vi "Fetch Control Method Info.vi"(6 "Parser Settings":T1, 8 "Error in":errorcluster caption="Error in (no error)", 10 "Dispatch (None)":T4, 11 "VI in":refnum<vi>) -> (0 "Error out":errorcluster, 3 "Method Spec Cluster":T5)   [LabVIEW 2023, in "VIDoc Parsing.lvlib"]
uses:
  VIDoc Parsing.lvlib
  TypeDefs/Method Spec Cluster.ctl
  TypeDefs/VI Type Extended Enum.ctl
  <vilib>/picture/picture.llb/imagedata.ctl
  TypeDefs/Class Dispatch Type Enum.ctl
  TypeDefs/Controls Info Cluster.ctl
  <vilib>/Utility/miscctls.llb/LVKeyTypeDef.ctl
  <vilib>/Utility/miscctls.llb/LVPointTypeDef.ctl
  Structure Reporter/Tree Cluster.ctl
  Settings/Parser Settings/Parser Settings Cluster.ctl
  Settings/Parser Settings/Draw Controls Cluster.ctl
  Settings/Parser Settings/Draw Option Enum.ctl
  Structure Reporter/Structure Reporter.lvlib
  Settings/Parser Settings/Parser Settings.lvclass
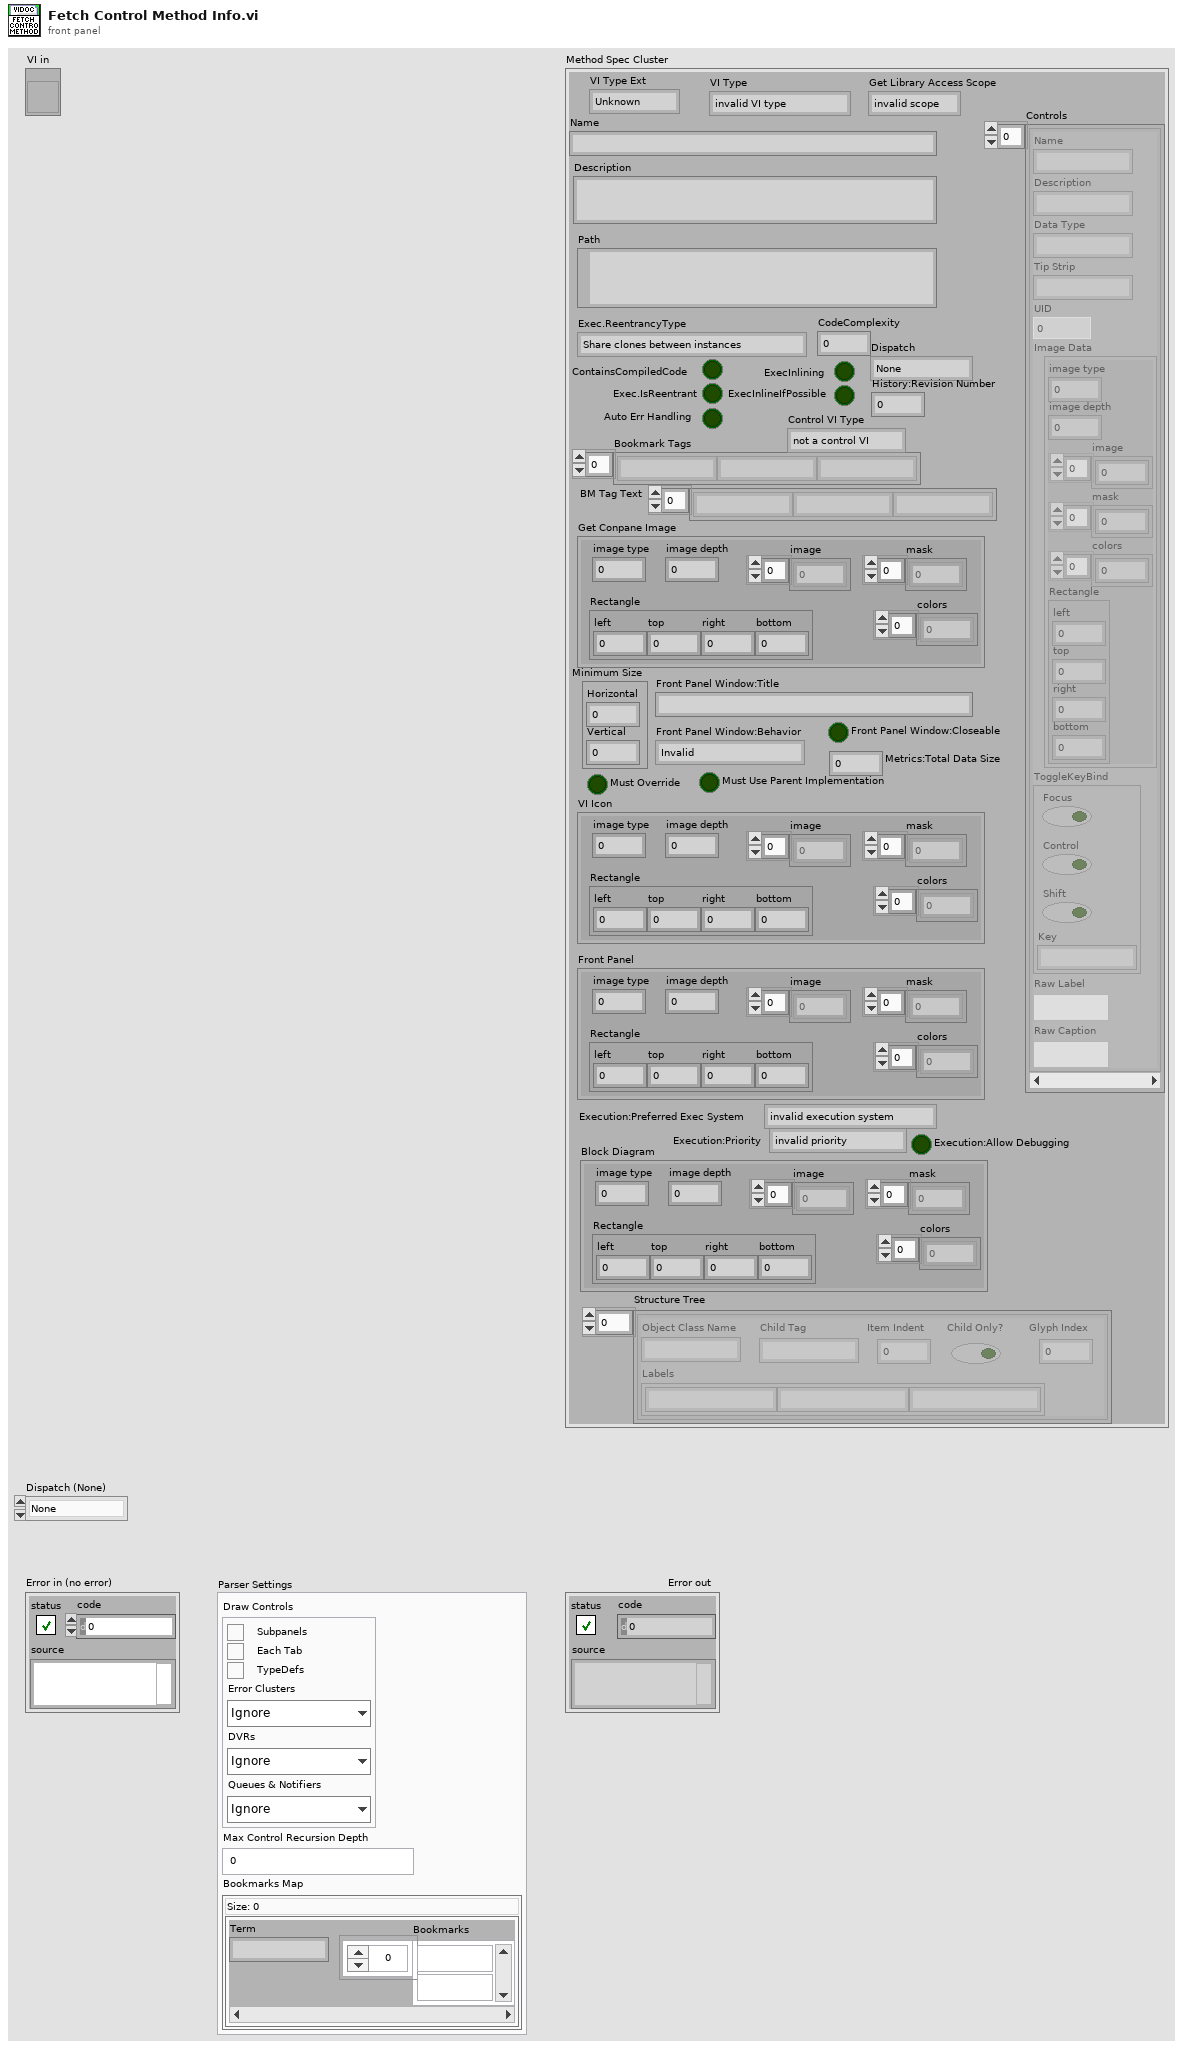
[diagram p1: front panel]
types:
  T1 = typedef "VIDoc Parsing.lvlib/Parser Settings.lvclass/Parser Settings Cluster.ctl" = cluster{"Draw Controls":T2, "Max Control Recursion Depth":i32, "Bookmarks Map":map{string, string[]}}
  T2 = typedef "VIDoc Parsing.lvlib/Parser Settings.lvclass/Draw Controls Cluster.ctl" = cluster{"Subpanels":bool, "Tabs":bool, "TypeDefs":bool, "Error Clusters":T3, "DVRs":T3, "Queues & Notifiers":T3}
  T3 = typedef "VIDoc Parsing.lvlib/Parser Settings.lvclass/Draw Option Enum.ctl" = enum16{"Ignore", "Draw", "Draw + Contents"}
  T4 = typedef "VIDoc Parsing.lvlib/Class Dispatch Type Enum.ctl" = enum16{"None", "Static", "Dynamic"}
  T5 = typedef "VIDoc Parsing.lvlib/Method Spec Cluster.ctl" = cluster{"VI Type Ext":T6, "Name":string, "Path":path, "Get Conpane Image":T7, "Description":string, "Get Library Access Scope":enum32{"invalid scope", "public", "private", "protected", "community"}, "Dispatch":T4, "ContainsCompiledCode":bool, "Exec.IsReentrant":bool, "Exec.ReentrancyType":enum16{"Share clones between instances", "Preallocate clone for each instance"}, "ExecInlining":bool, "ExecInlineIfPossible":bool, "Auto Err Handling":bool, "CodeComplexity":sgl, "Bookmark Tags":string[], "Control VI Type":enum32{"not a control VI", "control", "typedef", "strict typedef"}, "Controls":T8[], "VI Type":enum32{"invalid VI type", "Standard VI", "Control VI", "Global VI", "Polymorphic VI", "Configuration VI", "SubSystem", "Facade VI", "Method VI", "Statechart Diagram VI"}, "Minimum Size":T10, "Front Panel Window:Title":string, "Front Panel Window:Behavior":enum32{"Invalid", "Default", "Floating", "Floating/Auto-Hide", "Modal"}, "Front Panel Window:Closeable":bool, "Must Override":bool, "Must Use Parent Implementation":bool, "VI Icon":T7, "Front Panel":T7, "History:Revision Number":u32, "Metrics:Total Data Size":u32, "Execution:Allow Debugging":bool, "Execution:Preferred Exec System":enum32{"invalid execution system", "user interface", "standard", "instrument i/o", "data acquisition", "other 1", "other 2", "same as caller"}, "Execution:Priority":enum32{"invalid priority", "background priority", "normal priority", "above normal priority", "high priority", "time critical priority", "subroutine"}, "BM Tag Text":string[], "Block Diagram":T7, "Structure Tree":T11[]}
  T6 = typedef "VIDoc Parsing.lvlib/VI Type Extended Enum.ctl" = enum16{"Unknown", "Class Method", "Class Accessor Get", "Class Accessor Set", "Class Control", "Library Method", "Library Control", "VI", "Control"}
  T7 = typedef "imagedata.ctl" = cluster{"image type":i32, "image depth":i32, "image":u8[], "mask":u8[], "colors":u32[], "Rectangle":cluster{"left":i16, "top":i16, "right":i16, "bottom":i16}}
  T8 = typedef "VIDoc Parsing.lvlib/Controls Info Cluster.ctl" = cluster{"Name":string, "Description":string, "Data Type":string, "Tip Strip":string, "UID":i32, "Image Data":T7, "ToggleKeyBind":T9, "Raw Label":string, "Raw Caption":string}
  T9 = typedef "LVKeyTypeDef.ctl" = cluster{"Focus":bool, "Control":bool, "Shift":bool, "Key":string}
  T10 = typedef "LVPointTypeDef.ctl" = cluster{"Horizontal":i16, "Vertical":i16}
  T11 = typedef "VIDoc Parsing.lvlib/Structure Reporter.lvlib/Tree Cluster.ctl" = cluster{"Object Class Name":string, "Labels":string[], "Child Tag":string, "Item Indent":i32, "Child Only?":bool, "Glyph Index":i32}
  T12 = enum16{"Share clones between instances", "Preallocate clone for each instance"}
  T13 = enum32{"invalid scope", "public", "private", "protected", "community"}
  T14 = enum32{"invalid VI type", "Standard VI", "Control VI", "Global VI", "Polymorphic VI", "Configuration VI", "SubSystem", "Facade VI", "Method VI", "Statechart Diagram VI"}
  T15 = enum32{"not a control VI", "control", "typedef", "strict typedef"}
  T16 = enum32{"invalid execution system", "user interface", "standard", "instrument i/o", "data acquisition", "other 1", "other 2", "same as caller"}
  T17 = enum32{"invalid priority", "background priority", "normal priority", "above normal priority", "high priority", "time critical priority", "subroutine"}
  T18 = typedef "LVBookmarkInfoTypeDef.ctl" = cluster{"Bookmark ID":u32, "Bookmark Tag":string, "Label Text":string}[]
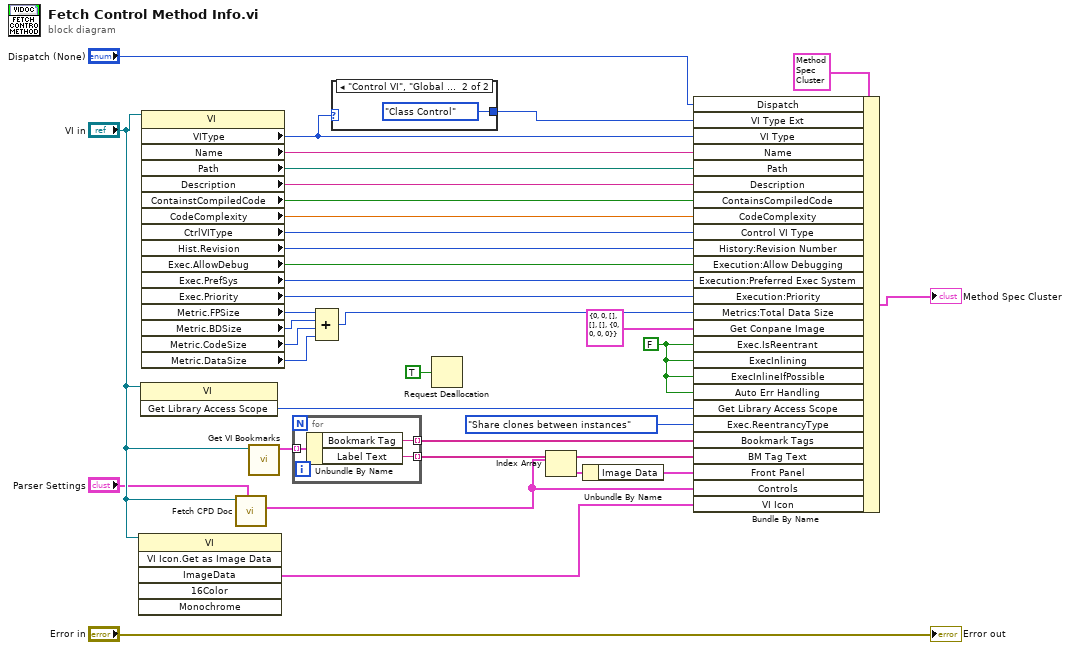
[diagram p0: block diagram]
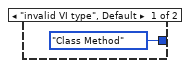
[diagram p2: hidden frame]
diagram:
  w8 = FALSE ("Exec.IsReentrant")
  n1 = invoke class="VI" method="VI Icon.Get as Image Data"(reference="VI in") -> ("ImageData"=w11:T7)  [unwired: 5 in, 5 out]
  n2 = invoke class="VI" method="Get Library Access Scope"(reference="VI in") -> ("Get Library Access Scope"=w6:T13)  [unwired: 2 in, 2 out]
  n3 = property class="VI"(reference="VI in") -> ("VIType"=w10:T14, "Name"=w30:string, "Path"=w25:path, "Description"=w20:string, "ContainstCompiledCode"=w19:bool, "CodeComplexity"=w18:sgl, "CtrlVIType"=w17:T15, "Hist.Revision"=w16:u32, "Exec.AllowDebug"=w15:bool, "Exec.PrefSys"=w14:T16, "Exec.Priority"=w13:T17, "Metric.FPSize"=w24:u32, "Metric.BDSize"=w23:u32, "Metric.CodeSize"=w22:u32, "Metric.DataSize"=w21:u32)  [unwired: 1 in, 2 out]
  n4 = call "Fetch CPD Doc.vi"("Parser Settings"="Parser Settings", "VI in"="VI in") -> ("Class Private Data"=w3:T8[])  [unwired: 8 in, 1 out]
  n5 = call "Get VI Bookmarks.vi"("VI in"="VI in") -> ("BookmarkInfo"=w27:T18)  [unwired: 9 in, 1 out]
  n6 = for {
    tunnel: w27 -> [w38] mode=indexing
    tunnel: [w37] -> w32 mode=indexing
    tunnel: [w36] -> w26 mode=indexing
    n7 = Unbundle By Name(w38) -> ("Bookmark Tag"=w37:string, "Label Text"=w36:string)
  }
  n8 = Compound Arithmetic op=ADD(w24, w23, w22, w21) -> (w12:u32)
  n9 = case shown="\"Control VI\", \"Global VI\"" w10 {
    tunnel: [VI_Type_Extended_Enum."Class Method" ("VI Type Ext") VI_Type_Extended_Enum."Class Control" ("VI Type Ext")] -> w34
    frame "invalid VI type", Default {
    }
    frame "Control VI", "Global VI" {
    }
  }
  n10 = Request Deallocation(TRUE ("flag")) -> ()
  n11 = Index Array(array=w3) -> (element=w2:T8)  [unwired: 1 in]
  n12 = Unbundle By Name(w2) -> ("Image Data"=w1:T7)
  n13 = Bundle By Name(cluster=T5 {"VI Type Ext"=enum."Unknown", "Name"="", "Path"=path "", "Get Conpane Image"={"image type"=0, "image depth"=0, "image"=[], "mask"=[], "colors"=[], "Rectangle"={"left"=0, "top"=0, "right"=0, "bottom"=0}}, "Description"="", "Get Library Access Scope"=enum."invalid scope", "Dispatch"=enum."None", "ContainsCompiledCode"=FALSE, "Exec.IsReentrant"=FALSE, "Exec.ReentrancyType"=enum."Share clones between instances", "ExecInlining"=FALSE, "ExecInlineIfPossible"=FALSE, "Auto Err Handling"=FALSE, "CodeComplexity"=0.0, "Bookmark Tags"=[], "Control VI Type"=enum."not a control VI", "Controls"=[], "VI Type"=enum."invalid VI type", "Minimum Size"={"Horizontal"=0, "Vertical"=0}, "Front Panel Window:Title"="", "Front Panel Window:Behavior"=enum."Invalid", "Front Panel Window:Closeable"=FALSE, "Must Override"=FALSE, "Must Use Parent Implementation"=FALSE, "VI Icon"={"image type"=0, "image depth"=0, "image"=[], "mask"=[], "colors"=[], "Rectangle"={"left"=0, "top"=0, "right"=0, "bottom"=0}}, "Front Panel"={"image type"=0, "image depth"=0, "image"=[], "mask"=[], "colors"=[], "Rectangle"={"left"=0, "top"=0, "right"=0, "bottom"=0}}, "History:Revision Number"=0, "Metrics:Total Data Size"=0, "Execution:Allow Debugging"=FALSE, "Execution:Preferred Exec System"=enum."invalid execution system", "Execution:Priority"=enum."invalid priority", "BM Tag Text"=[], "Block Diagram"={"image type"=0, "image depth"=0, "image"=[], "mask"=[], "colors"=[], "Rectangle"={"left"=0, "top"=0, "right"=0, "bottom"=0}}, "Structure Tree"=[]}, "Dispatch"="Dispatch (None)", "VI Type Ext"=w34, "VI Type"=w10, "Name"=w30, "Path"=w25, "Description"=w20, "ContainsCompiledCode"=w19, "CodeComplexity"=w18, "Control VI Type"=w17, "History:Revision Number"=w16, "Execution:Allow Debugging"=w15, "Execution:Preferred Exec System"=w14, "Execution:Priority"=w13, "Metrics:Total Data Size"=w12, "Get Conpane Image"=T7 {"image type"=0, "image depth"=0, "image"=[], "mask"=[], "colors"=[], "Rectangle"={"left"=0, "top"=0, "right"=0, "bottom"=0}}, "Exec.IsReentrant"=w8, "ExecInlining"=w8, "ExecInlineIfPossible"=w8, "Auto Err Handling"=w8, "Get Library Access Scope"=w6, "Exec.ReentrancyType"=T12."Share clones between instances", "Bookmark Tags"=w32, "BM Tag Text"=w26, "Front Panel"=w1, "Controls"=w3, "VI Icon"=w11) -> (→"Method Spec Cluster":T5)
  "Error out" <- "Error in"
